vi "freq_scan_FRXYPPhase_6_23_2025.vi"() -> ()   [LabVIEW 2010]
uses:
  <vilib>/Utility/file.llb/Write To Spreadsheet File (string).vi
  <vilib>/Utility/file.llb/Write To Spreadsheet File (DBL).vi
panel:
  in  "DC offset":ext format="%.3f"
  in  "?":enum32{"Amp v.s Freq", "X & Y v.s Freq"}(tab)
  in  "Unit":i8=1 min=0 max=2 step=1
  in  "Start Frequency":dbl=1.635 min=0.0 format="%.3f"
  in  "End Frequency":dbl=3.0 min=0.0 format="%.3f"
  in  "Step in Hz":dbl=1.0 min=0.0 format="%.2f"
  in  "Step interval in ms":u32=500
  in  "Sensitivity":u16(ring)=20 items=["2 nV/fA", "5 nV/fA", "10 nV/fA", "20 nV/fA", "50 nV/fA", "100 nV/fA", "200 nV/fA", "500 nV/fA", "1 uV/pA", "2 uV/pA", "5 uV/pA", "10 uV/pA", "20 uV/pA", "50 uV/pA", "100 uV/pA", "200 uV/pA", "500 uV/pA", "1 mV/nA", "2 mV/nA", "5 mV/nA", "10 mV/nA", "20 mV/nA", "50 mV/nA", "100 mV/nA", "200 mV/nA", "500 mV/nA", "1 V/uA"]
  in  "Detection Bandwidth":u16(ring)=7 items=["25 kHz", "8.33 kHz", "2.50 kHz", "833 Hz", "250 Hz", "83.3 Hz", "25 Hz", "8.33 Hz", "2.50 Hz", "0.833 Hz", "0.250 Hz", "0.0833 Hz", "0.025 Hz"]
  in  "Phase":dbl
  in  "Driving amp (0 Vrms:0)":cluster{ext, i32}={0.05, 0} {"?" items=["Vrms", "Vpp", "dBm"]; "?" format="%.3f"}
  out "freq":string="22749"
  out "amp":string="0.000175477"
  out "Amp vs Freq":cluster{dbl, dbl}[](graph)=[{21250.0, 6.10356e-05}, {21252.3, 0.000320436}, {21254.6, 0.00027466}, {21256.899999999998, 0.000175477}, {21259.199999999997, 0.000297548}, {21261.499999999996, 0.000343325}, {21263.799999999996, 0.000251772}, {21266.099999999995, 0.00027466}, {21268.399999999994, 0.000297548}, {21270.699999999993, 6.8665e-05}, {21272.999999999993, 0.000251772}, {21275.299999999992, 9.91826e-05}, {21277.59999999999, 0.000251772}, {21279.89999999999, 0.00027466}, {21282.19999999999, 3.81472e-05}, {21284.49999999999, 0.000366213}, {21286.79999999999, 0.00013733}, {21289.099999999988, 0.000144959}, {21291.399999999987, 0.000221253}, {21293.699999999986, 0.000328066}, {21295.999999999985, 0.000259401}, {21298.299999999985, 0.000236512}, {21300.599999999984, 0.000228883}, {21302.899999999983, 0.000167848}, {21305.199999999983, 0.000297548}, {21307.49999999998, 0.000167848}, {21309.79999999998, 0.000213624}, {21312.09999999998, 0.000228883}, {21314.39999999998, 0.000289919}, {21316.69999999998, 0.00013733}, {21318.999999999978, 6.8665e-05}, {21321.299999999977, 0.000366213}, {21323.599999999977, 7.62944e-05}, {21325.899999999976, 0.000228883}, {21328.199999999975, 0.000381472}, {21330.499999999975, 0.000259401}, {21332.799999999974, 0.000167848}, {21335.099999999973, 0.000175477}, {21337.399999999972, 0.000343325}, {21339.69999999997, 0.000312807}, {21341.99999999997, 6.10356e-05}, {21344.29999999997, 0.000205995}, {21346.59999999997, 0.000129701}, {21348.89999999997, 0.000343325}, {21351.199999999968, 9.91826e-05}, {21353.499999999967, 0.000434877}, {21355.799999999967, 0.000373842}, {21358.099999999966, 0.000251772}, {21360.399999999965, 0.000328066}, {21362.699999999964, 0.000122071}, {21364.999999999964, 0.00039673}, {21367.299999999963, 0.000244142}, {21369.599999999962, 0.000366213}, {21371.89999999996, 0.000381472}, {21374.19999999996, 0.000350954}, {21376.49999999996, 0.000289919}, {21378.79999999996, 4.57766e-05}, {21381.09999999996, 0.000373842}, {21383.399999999958, 0.000312807}, {21385.699999999957, 9.91826e-05}, {21387.999999999956, 0.000114441}, {21390.299999999956, 0.000305178}, {21392.599999999955, 0.000175477}, {21394.899999999954, 0.000205995}, {21397.199999999953, 0.000190736}, {21399.499999999953, 0.00040436}, {21401.799999999952, 0.00013733}, {21404.09999999995, 9.91826e-05}, {21406.39999999995, 0.000320436}, {21408.69999999995, 0.000160218}, {21410.99999999995, 0.000419619}, {21413.29999999995, 0.000152589}, {21415.599999999948, 0.000320436}, {21417.899999999947, 0.000175477}, {21420.199999999946, 0.000183106}, {21422.499999999945, 9.91826e-05}, {21424.799999999945, 0.000152589}, {21427.099999999944, 0.000411989}, {21429.399999999943, 0.000366213}, {21431.699999999943, 0.000457766}, {21433.99999999994, 0.00040436}, {21436.29999999994, 0.000419619}, {21438.59999999994, 0.000259401}, {21440.89999999994, 0.000457766}, {21443.19999999994, 0.000205995}, {21445.499999999938, 0.000419619}, {21447.799999999937, 0.000106812}, {21450.099999999937, 0.000305178}, {21452.399999999936, 0.000267031}, {21454.699999999935, 0.00040436}, {21456.999999999935, 0.000381472}, {21459.299999999934, 0.000366213}, {21461.599999999933, 0.000411989}, {21463.899999999932, 0.000160218}, {21466.19999999993, 0.000259401}, {21468.49999999993, 0.000205995}, {21470.79999999993, 0.000282289}, {21473.09999999993, 0.000335695}, {21475.39999999993, 0.000328066}, {21477.699999999928, 0.000175477}, {21479.999999999927, 0.000419619}, {21482.299999999927, 0.00040436}, {21484.599999999926, 0.00040436}, {21486.899999999925, 0.000259401}, {21489.199999999924, 0.000236512}, {21491.499999999924, 0.000427248}, {21493.799999999923, 0.00039673}, {21496.099999999922, 0.000236512}, {21498.39999999992, 0.000373842}, {21500.69999999992, 0.000221253}, {21502.99999999992, 0.000465395}, {21505.29999999992, 0.000419619}, {21507.59999999992, 0.000320436}, {21509.899999999918, 0.000190736}, {21512.199999999917, 0.000465395}, {21514.499999999916, 0.000343325}, {21516.799999999916, 0.000473024}, {21519.099999999915, 0.000282289}, {21521.399999999914, 0.000419619}, {21523.699999999913, 0.000335695}, {21525.999999999913, 0.000411989}, {21528.299999999912, 0.000267031}, {21530.59999999991, 0.000289919}, {21532.89999999991, 0.000389101}, {21535.19999999991, 0.000236512}, {21537.49999999991, 0.000221253}, {21539.79999999991, 0.000450136}, {21542.099999999908, 0.000541691}, {21544.399999999907, 0.00039673}, {21546.699999999906, 0.000312807}, {21548.999999999905, 0.000205995}, {21551.299999999905, 0.000534061}, {21553.599999999904, 0.000442507}, {21555.899999999903, 0.000457766}, {21558.199999999903, 0.000434877}, {21560.4999999999, 0.000419619}, {21562.7999999999, 0.00039673}, {21565.0999999999, 0.000350954}, {21567.3999999999, 0.000534061}, {21569.6999999999, 0.000534061}, {21571.999999999898, 0.000328066}, {21574.299999999897, 0.000267031}, {21576.599999999897, 0.000564579}, {21578.899999999896, 0.000251772}, {21581.199999999895, 0.000541691}, {21583.499999999894, 0.000564579}, {21585.799999999894, 0.000579838}, {21588.099999999893, 0.000366213}, {21590.399999999892, 0.000343325}, {21592.69999999989, 0.000579838}, {21594.99999999989, 0.000579838}, {21597.29999999989, 0.000633243}, {21599.59999999989, 0.000480654}, {21601.89999999989, 0.000511173}, {21604.199999999888, 0.000488285}, {21606.499999999887, 0.000656132}, {21608.799999999886, 0.000366213}, {21611.099999999886, 0.000419619}, {21613.399999999885, 0.00067902}, {21615.699999999884, 0.000366213}, {21617.999999999884, 0.00039673}, {21620.299999999883, 0.00067139}, {21622.599999999882, 0.000633243}, {21624.89999999988, 0.000495914}, {21627.19999999988, 0.000427248}, {21629.49999999988, 0.00055695}, {21631.79999999988, 0.000427248}, {21634.09999999988, 0.00040436}, {21636.399999999878, 0.000579838}, {21638.699999999877, 0.000526432}, {21640.999999999876, 0.00067139}, {21643.299999999876, 0.000473024}, {21645.599999999875, 0.000610355}, {21647.899999999874, 0.000511173}, {21650.199999999873, 0.000526432}, {21652.499999999873, 0.000762943}, {21654.799999999872, 0.000762943}, {21657.09999999987, 0.000785831}, {21659.39999999987, 0.000595096}, {21661.69999999987, 0.000740055}, {21663.99999999987, 0.00080109}, {21666.29999999987, 0.000747684}, {21668.599999999868, 0.000564579}, {21670.899999999867, 0.000732426}, {21673.199999999866, 0.000602726}, {21675.499999999865, 0.00080872}, {21677.799999999865, 0.000656132}, {21680.099999999864, 0.000938419}, {21682.399999999863, 0.000846867}, {21684.699999999862, 0.000587467}, {21686.99999999986, 0.000709537}, {21689.29999999986, 0.000869755}, {21691.59999999986, 0.00067902}, {21693.89999999986, 0.000900272}, {21696.19999999986, 0.00067902}, {21698.499999999858, 0.000701908}, {21700.799999999857, 0.000999458}, {21703.099999999857, 0.000968937}, {21705.399999999856, 0.000885013}, {21707.699999999855, 0.00102998}, {21709.999999999854, 0.000839237}, {21712.299999999854, 0.000968937}, {21714.599999999853, 0.000823978}, {21716.899999999852, 0.000968937}, {21719.19999999985, 0.000991829}, {21721.49999999985, 0.00115968}, {21723.79999999985, 0.00114442}, {21726.09999999985, 0.00115968}, {21728.39999999985, 0.000999458}, {21730.699999999848, 0.000999458}, {21732.999999999847, 0.00110627}, {21735.299999999846, 0.000999458}, {21737.599999999846, 0.000938419}, {21739.899999999845, 0.00106812}, {21742.199999999844, 0.00126649}, {21744.499999999844, 0.00119019}, {21746.799999999843, 0.00110627}, {21749.099999999842, 0.00141145}, {21751.39999999984, 0.00105286}, {21753.69999999984, 0.00122071}, {21755.99999999984, 0.00141145}, {21758.29999999984, 0.001297}, {21760.59999999984, 0.00121308}, {21762.899999999838, 0.00139619}, {21765.199999999837, 0.00127412}, {21767.499999999836, 0.0014267}, {21769.799999999836, 0.00122071}, {21772.099999999835, 0.00154115}, {21774.399999999834, 0.00148011}, {21776.699999999833, 0.00144959}, {21778.999999999833, 0.00144196}, {21781.299999999832, 0.00157929}, {21783.59999999983, 0.00154877}, {21785.89999999983, 0.0016327}, {21788.19999999983, 0.0013733}, {21790.49999999983, 0.0016327}, {21792.79999999983, 0.00154115}, {21795.099999999828, 0.00177003}, {21797.399999999827, 0.00159455}, {21799.699999999826, 0.00157929}, {21801.999999999825, 0.0018921}, {21804.299999999825, 0.00180817}, {21806.599999999824, 0.00199129}, {21808.899999999823, 0.0018158}, {21811.199999999822, 0.00175477}, {21813.49999999982, 0.0020218}, {21815.79999999982, 0.00197603}, {21818.09999999982, 0.00199129}, {21820.39999999982, 0.00189973}, {21822.69999999982, 0.0019455}, {21824.999999999818, 0.00215913}, {21827.299999999817, 0.00206758}, {21829.599999999817, 0.0020981}, {21831.899999999816, 0.00238039}, {21834.199999999815, 0.00229646}, {21836.499999999814, 0.00234987}, {21838.799999999814, 0.00221254}, {21841.099999999813, 0.00251009}, {21843.399999999812, 0.00250246}, {21845.69999999981, 0.00238802}, {21847.99999999981, 0.00263979}, {21850.29999999981, 0.00263979}, {21852.59999999981, 0.00271608}, {21854.89999999981, 0.00264741}, {21857.199999999808, 0.00276949}, {21859.499999999807, 0.00289918}, {21861.799999999806, 0.00279237}, {21864.099999999806, 0.00311281}, {21866.399999999805, 0.00309755}, {21868.699999999804, 0.003006}, {21870.999999999804, 0.00324251}, {21873.299999999803, 0.00321962}, {21875.599999999802, 0.00341035}, {21877.8999999998, 0.00349428}, {21880.1999999998, 0.00351717}, {21882.4999999998, 0.00358583}, {21884.7999999998, 0.00382997}, {21887.0999999998, 0.00371553}, {21889.399999999798, 0.00389864}, {21891.699999999797, 0.0040665}, {21893.999999999796, 0.00415805}, {21896.299999999796, 0.00434116}, {21898.599999999795, 0.00444797}, {21900.899999999794, 0.00473788}, {21903.199999999793, 0.00467685}, {21905.499999999793, 0.00499728}, {21907.799999999792, 0.00508884}, {21910.09999999979, 0.00527957}, {21912.39999999979, 0.00547031}, {21914.69999999979, 0.00560763}, {21916.99999999979, 0.0060654}, {21919.29999999979, 0.00611117}, {21921.599999999788, 0.00637057}, {21923.899999999787, 0.00639346}, {21926.199999999786, 0.00661471}, {21928.499999999785, 0.007103}, {21930.799999999785, 0.00733188}, {21933.099999999784, 0.00738528}, {21935.399999999783, 0.00758365}, {21937.699999999782, 0.00788122}, {21939.99999999978, 0.00812536}, {21942.29999999978, 0.00841528}, {21944.59999999978, 0.00881201}, {21946.89999999978, 0.00908667}, {21949.19999999978, 0.00920874}, {21951.499999999778, 0.00949866}, {21953.799999999777, 0.00976568}, {21956.099999999777, 0.00971991}, {21958.399999999776, 0.0100632}, {21960.699999999775, 0.00996405}, {21962.999999999774, 0.0100861}, {21965.299999999774, 0.0105668}, {21967.599999999773, 0.0105591}, {21969.899999999772, 0.0102311}, {21972.19999999977, 0.0103455}, {21974.49999999977, 0.0102921}, {21976.79999999977, 0.00994879}, {21979.09999999977, 0.0101548}, {21981.39999999977, 0.00997931}, {21983.699999999768, 0.00973517}, {21985.999999999767, 0.00996405}, {21988.299999999766, 0.00971991}, {21990.599999999766, 0.00950629}, {21992.899999999765, 0.00929266}, {21995.199999999764, 0.00900275}, {21997.499999999764, 0.00892645}, {21999.799999999763, 0.00866705}, {22002.099999999762, 0.00841528}, {22004.39999999976, 0.00823981}, {22006.69999999976, 0.00823218}, {22008.99999999976, 0.00795752}, {22011.29999999976, 0.00795752}, {22013.59999999976, 0.00768283}, {22015.899999999758, 0.00753024}, {22018.199999999757, 0.00725558}, {22020.499999999756, 0.00695804}, {22022.799999999756, 0.00716403}, {22025.099999999755, 0.00704196}, {22027.399999999754, 0.00678256}, {22029.699999999753, 0.00693515}, {22031.999999999753, 0.00656894}, {22034.299999999752, 0.00638583}, {22036.59999999975, 0.00646213}, {22038.89999999975, 0.00610355}, {22041.19999999975, 0.00594333}, {22043.49999999975, 0.00572208}, {22045.79999999975, 0.00559238}, {22048.099999999748, 0.00569919}, {22050.399999999747, 0.00543979}, {22052.699999999746, 0.00527957}, {22054.999999999745, 0.00548556}, {22057.299999999745, 0.00524142}, {22059.599999999744, 0.00514987}, {22061.899999999743, 0.00496677}, {22064.199999999742, 0.00514224}, {22066.49999999974, 0.00485232}, {22068.79999999974, 0.00475314}, {22071.09999999974, 0.00464633}, {22073.39999999974, 0.004509}, {22075.69999999974, 0.00459293}, {22077.999999999738, 0.00452426}, {22080.299999999737, 0.00453189}, {22082.599999999737, 0.00426486}, {22084.899999999736, 0.00421146}, {22087.199999999735, 0.00408939}, {22089.499999999734, 0.00405887}, {22091.799999999734, 0.0039902}, {22094.099999999733, 0.0038376}, {22096.399999999732, 0.00404361}, {22098.69999999973, 0.00389864}, {22100.99999999973, 0.00384523}, {22103.29999999973, 0.00360109}, {22105.59999999973, 0.00365449}, {22107.89999999973, 0.00374605}, {22110.199999999728, 0.00364687}, {22112.499999999727, 0.00337984}, {22114.799999999726, 0.00334169}, {22117.099999999726, 0.00337984}, {22119.399999999725, 0.0035782}, {22121.699999999724, 0.0034485}, {22123.999999999724, 0.00320436}, {22126.299999999723, 0.00312807}, {22128.599999999722, 0.00314333}, {22130.89999999972, 0.00306703}, {22133.19999999972, 0.00307466}, {22135.49999999972, 0.00319673}, {22137.79999999972, 0.00307466}, {22140.09999999972, 0.00303651}, {22142.399999999718, 0.00295259}, {22144.699999999717, 0.00297548}, {22146.999999999716, 0.00293733}, {22149.299999999716, 0.00272371}, {22151.599999999715, 0.00291444}, {22153.899999999714, 0.00256349}, {22156.199999999713, 0.00259401}, {22158.499999999713, 0.00244142}, {22160.799999999712, 0.00264741}, {22163.09999999971, 0.00246431}, {22165.39999999971, 0.00253297}, {22167.69999999971, 0.00250246}, {22169.99999999971, 0.00232698}, {22172.29999999971, 0.0024872}, {22174.599999999708, 0.00251772}, {22176.899999999707, 0.00232698}, {22179.199999999706, 0.00205232}, {22181.499999999705, 0.00231935}, {22183.799999999705, 0.00214387}, {22186.099999999704, 0.00216676}, {22188.399999999703, 0.00218202}, {22190.699999999702, 0.00189973}, {22192.9999999997, 0.0021515}, {22195.2999999997, 0.00204469}, {22197.5999999997, 0.00198366}, {22199.8999999997, 0.00209047}, {22202.1999999997, 0.00180054}, {22204.499999999698, 0.00198366}, {22206.799999999697, 0.00195314}, {22209.099999999697, 0.00167847}, {22211.399999999696, 0.00170136}, {22213.699999999695, 0.00182343}, {22215.999999999694, 0.00162507}, {22218.299999999694, 0.00154115}, {22220.599999999693, 0.00186921}, {22222.899999999692, 0.001503}, {22225.19999999969, 0.00157166}, {22227.49999999969, 0.00162507}, {22229.79999999969, 0.00167084}, {22232.09999999969, 0.00130463}, {22234.39999999969, 0.00153352}, {22236.699999999688, 0.00160981}, {22238.999999999687, 0.00147248}, {22241.299999999686, 0.00160218}, {22243.599999999686, 0.00138093}, {22245.899999999685, 0.00153352}, {22248.199999999684, 0.00130463}, {22250.499999999683, 0.00126649}, {22252.799999999683, 0.00146485}, {22255.099999999682, 0.00121308}, {22257.39999999968, 0.00131989}, {22259.69999999968, 0.00119019}, {22261.99999999968, 0.00121308}, {22264.29999999968, 0.00110627}, {22266.59999999968, 0.00105286}, {22268.899999999678, 0.00122071}, {22271.199999999677, 0.00130463}, {22273.499999999676, 0.00130463}, {22275.799999999675, 0.00112153}, {22278.099999999675, 0.0011673}, {22280.399999999674, 0.00104523}, {22282.699999999673, 0.00134278}, {22284.999999999673, 0.00112916}, {22287.299999999672, 0.00126649}, {22289.59999999967, 0.00122071}, {22291.89999999967, 0.00103761}, {22294.19999999967, 0.00120545}, {22296.49999999967, 0.00128175}, {22298.79999999967, 0.00121308}, {22301.099999999667, 0.00110627}, {22303.399999999667, 0.00093079}, {22305.699999999666, 0.000953678}, {22307.999999999665, 0.0011673}, {22310.299999999665, 0.00110627}, {22312.599999999664, 0.00110627}, {22314.899999999663, 0.00121308}, {22317.199999999662, 0.00113679}, {22319.49999999966, 0.00117493}, {22321.79999999966, 0.00120545}, {22324.09999999966, 0.000961307}, {22326.39999999966, 0.000946049}, {22328.69999999966, 0.00128938}, {22330.999999999658, 0.00104523}, {22333.299999999657, 0.00102235}, {22335.599999999657, 0.00115968}, {22337.899999999656, 0.0012436}, {22340.199999999655, 0.00121308}, {22342.499999999654, 0.00120545}, {22344.799999999654, 0.00097657}, {22347.099999999653, 0.00108338}, {22349.399999999652, 0.00114442}, {22351.69999999965, 0.0011673}, {22353.99999999965, 0.00105286}, {22356.29999999965, 0.00097657}, {22358.59999999965, 0.00103761}, {22360.89999999965, 0.00131989}, {22363.199999999648, 0.0011673}, {22365.499999999647, 0.00127412}, {22367.799999999646, 0.00108338}, {22370.099999999646, 0.00121308}, {22372.399999999645, 0.00100709}, {22374.699999999644, 0.000999458}, {22376.999999999643, 0.00119019}, {22379.299999999643, 0.00119019}, {22381.599999999642, 0.00109101}, {22383.89999999964, 0.00125123}, {22386.19999999964, 0.00128175}, {22388.49999999964, 0.00105286}, {22390.79999999964, 0.00097657}, {22393.09999999964, 0.00130463}, {22395.399999999638, 0.00109864}, {22397.699999999637, 0.00104523}, {22399.999999999636, 0.00125123}, {22402.299999999635, 0.000869755}, {22404.599999999635, 0.00106812}, {22406.899999999634, 0.00117493}, {22409.199999999633, 0.000938419}, {22411.499999999633, 0.00122071}, {22413.799999999632, 0.00093079}, {22416.09999999963, 0.00107575}, {22418.39999999963, 0.00101472}, {22420.69999999963, 0.0011673}, {22422.99999999963, 0.00100709}, {22425.29999999963, 0.00118256}, {22427.599999999627, 0.00113679}, {22429.899999999627, 0.00101472}, {22432.199999999626, 0.00109101}, {22434.499999999625, 0.00112916}, {22436.799999999625, 0.00092316}, {22439.099999999624, 0.000839237}, {22441.399999999623, 0.00128175}, {22443.699999999622, 0.00121308}, {22445.99999999962, 0.00105286}, {22448.29999999962, 0.00109864}, {22450.59999999962, 0.00110627}, {22452.89999999962, 0.000823978}, {22455.19999999962, 0.000854496}, {22457.499999999618, 0.00103761}, {22459.799999999617, 0.00105286}, {22462.099999999617, 0.00097657}, {22464.399999999616, 0.000999458}, {22466.699999999615, 0.00102998}, {22468.999999999614, 0.000793461}, {22471.299999999614, 0.000732426}, {22473.599999999613, 0.00097657}, {22475.899999999612, 0.00102235}, {22478.19999999961, 0.000915531}, {22480.49999999961, 0.00097657}, {22482.79999999961, 0.000907902}, {22485.09999999961, 0.000823978}, {22487.39999999961, 0.00092316}, {22489.699999999608, 0.000831608}, {22491.999999999607, 0.000892643}, {22494.299999999606, 0.000732426}, {22496.599999999606, 0.000839237}, {22498.899999999605, 0.000709537}, {22501.199999999604, 0.000892643}, {22503.499999999603, 0.000793461}, {22505.799999999603, 0.000793461}, {22508.099999999602, 0.000854496}, {22510.3999999996, 0.000740055}, {22512.6999999996, 0.000877384}, {22514.9999999996, 0.000877384}, {22517.2999999996, 0.000526432}, {22519.5999999996, 0.000610355}, {22521.899999999598, 0.000770573}, {22524.199999999597, 0.000503544}, {22526.499999999596, 0.000816349}, {22528.799999999595, 0.000534061}, {22531.099999999595, 0.000717167}, {22533.399999999594, 0.000625614}, {22535.699999999593, 0.000656132}, {22537.999999999593, 0.000663761}, {22540.29999999959, 0.000434877}, {22542.59999999959, 0.000625614}, {22544.89999999959, 0.000473024}, {22547.19999999959, 0.000442507}, {22549.49999999959, 0.000717167}, {22551.799999999588, 0.00080109}, {22554.099999999587, 0.000350954}, {22556.399999999587, 0.000610355}, {22558.699999999586, 0.000526432}, {22560.999999999585, 0.000656132}, {22563.299999999585, 0.000633243}, {22565.599999999584, 0.000473024}, {22567.899999999583, 0.000328066}, {22570.199999999582, 0.00067139}, {22572.49999999958, 0.000564579}, {22574.79999999958, 0.000701908}, {22577.09999999958, 0.000526432}, {22579.39999999958, 0.000480654}, {22581.69999999958, 0.000656132}, {22583.999999999578, 0.00054932}, {22586.299999999577, 0.000381472}, {22588.599999999577, 0.000350954}, {22590.899999999576, 0.000511173}, {22593.199999999575, 0.000373842}, {22595.499999999574, 0.00027466}, {22597.799999999574, 0.000541691}, {22600.099999999573, 0.000663761}, {22602.399999999572, 0.000366213}, {22604.69999999957, 0.000564579}, {22606.99999999957, 0.00027466}, {22609.29999999957, 0.000511173}, {22611.59999999957, 0.00055695}, {22613.89999999957, 0.000312807}, {22616.199999999568, 0.000473024}, {22618.499999999567, 0.000473024}, {22620.799999999566, 0.000572208}, {22623.099999999566, 0.000465395}, {22625.399999999565, 0.000579838}, {22627.699999999564, 0.000465395}, {22629.999999999563, 0.000473024}, {22632.299999999563, 0.000427248}, {22634.599999999562, 0.00039673}, {22636.89999999956, 0.000480654}, {22639.19999999956, 0.000465395}, {22641.49999999956, 0.000534061}, {22643.79999999956, 0.000518803}, {22646.09999999956, 0.000289919}, {22648.399999999558, 0.000442507}, {22650.699999999557, 0.000541691}, {22652.999999999556, 0.000526432}, {22655.299999999555, 0.000534061}, {22657.599999999555, 0.000473024}, {22659.899999999554, 0.000457766}, {22662.199999999553, 0.000167848}, {22664.499999999553, 0.000259401}, {22666.79999999955, 0.000480654}, {22669.09999999955, 0.000175477}, {22671.39999999955, 0.00040436}, {22673.69999999955, 0.000221253}, {22675.99999999955, 0.000457766}, {22678.299999999548, 0.000518803}, {22680.599999999547, 0.000312807}, {22682.899999999547, 0.000312807}, {22685.199999999546, 0.000427248}, {22687.499999999545, 0.000366213}, {22689.799999999545, 0.000473024}, {22692.099999999544, 0.000473024}, {22694.399999999543, 0.00040436}, {22696.699999999542, 0.000450136}, {22698.99999999954, 0.000144959}, {22701.29999999954, 0.000228883}, {22703.59999999954, 0.000457766}, {22705.89999999954, 0.000144959}, {22708.19999999954, 8.39238e-05}, {22710.499999999538, 0.000411989}, {22712.799999999537, 0.000442507}, {22715.099999999537, 0.000228883}, {22717.399999999536, 0.000465395}, {22719.699999999535, 0.000259401}, {22721.999999999534, 0.000389101}, {22724.299999999534, 0.000503544}, {22726.599999999533, 0.000183106}, {22728.899999999532, 0.000289919}, {22731.19999999953, 0.00013733}, {22733.49999999953, 0.000244142}, {22735.79999999953, 0.000305178}, {22738.09999999953, 0.000259401}, {22740.39999999953, 0.000427248}, {22742.699999999528, 0.000221253}, {22744.999999999527, 9.91826e-05}, {22747.299999999526, 0.000175477}]
  out "Waveform Chart":cluster{dbl, dbl}(graph)
  in  "Path":path
  in  "On/Off":bool=TRUE
  # "Make sure to set DS345's GPIB address to 19.\nMake sure to set SR830's GPIB address to 8."
  # "0: Hz\n1: kHz\n2: MHz"
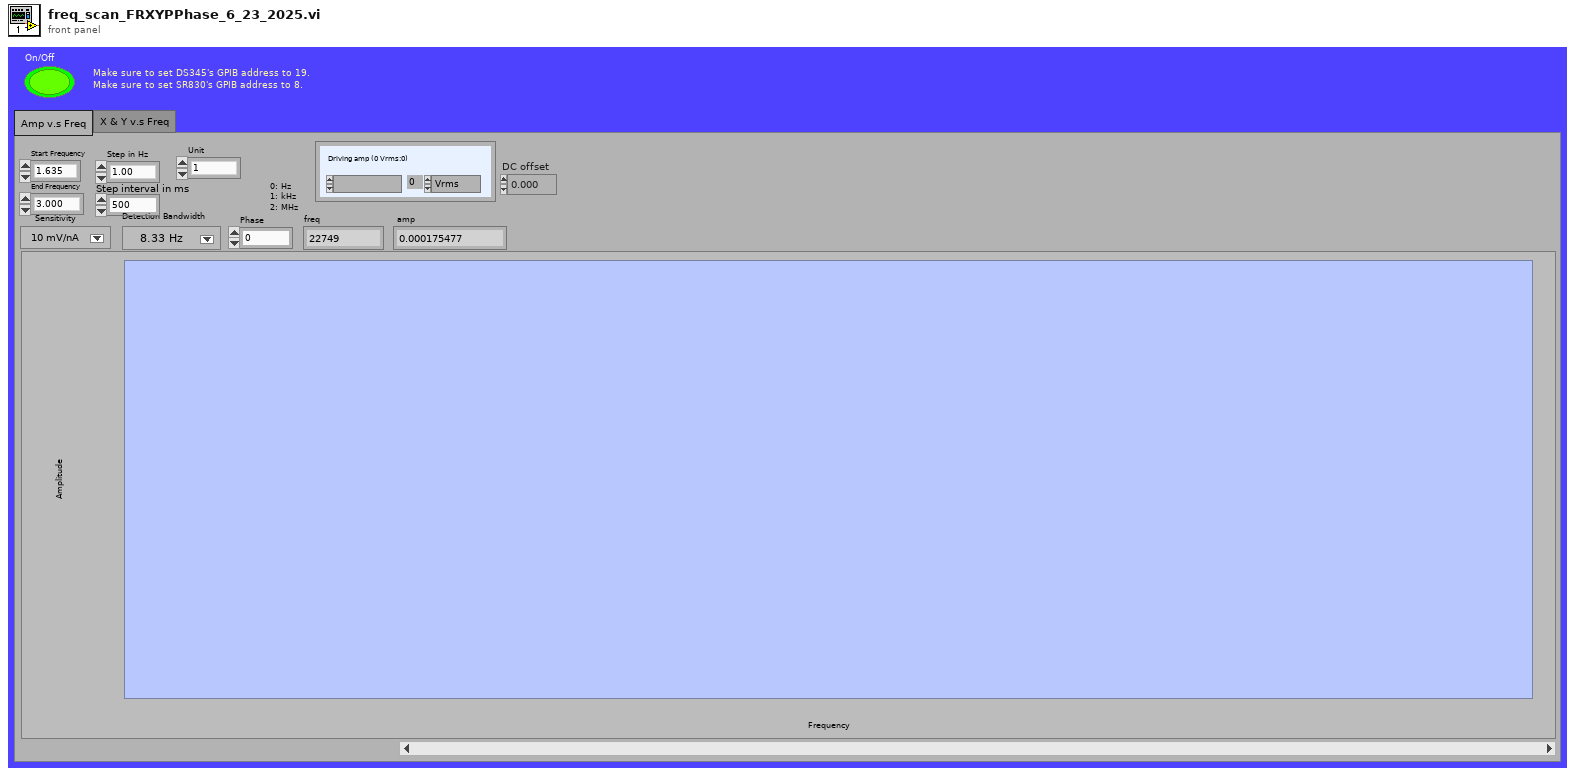
[diagram p1: front panel]
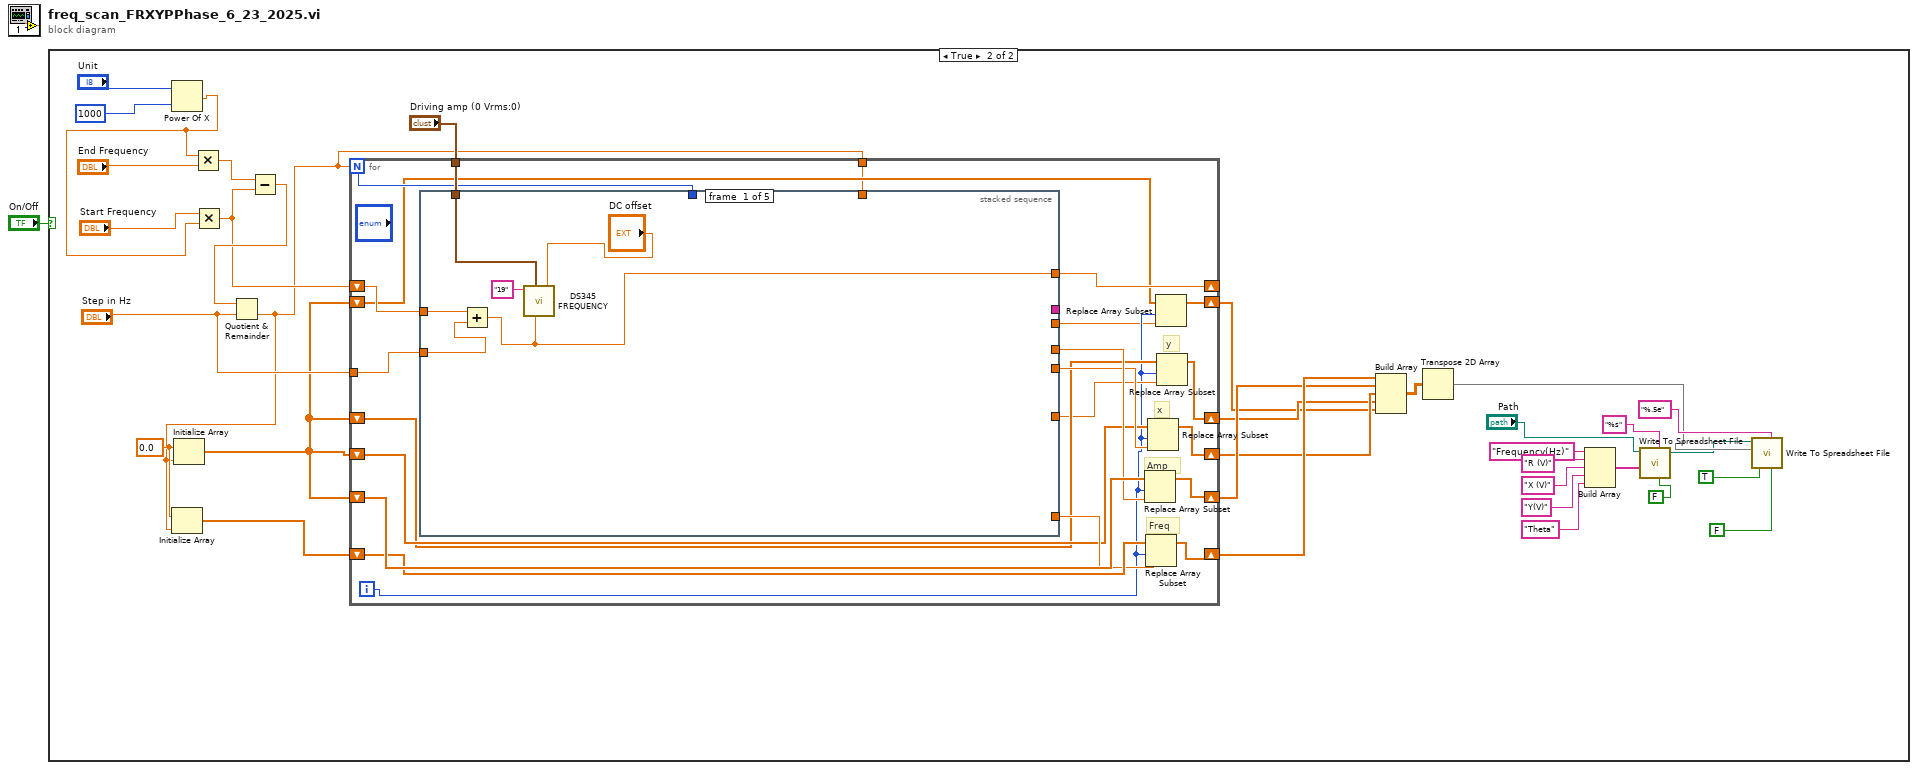
[diagram p0: block diagram]
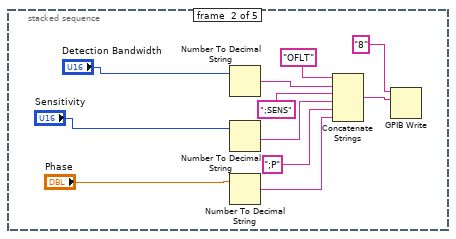
[diagram p3: hidden frame]
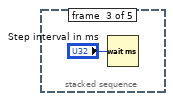
[diagram p4: hidden frame]
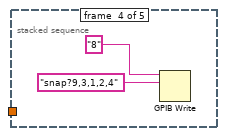
[diagram p5: hidden frame]
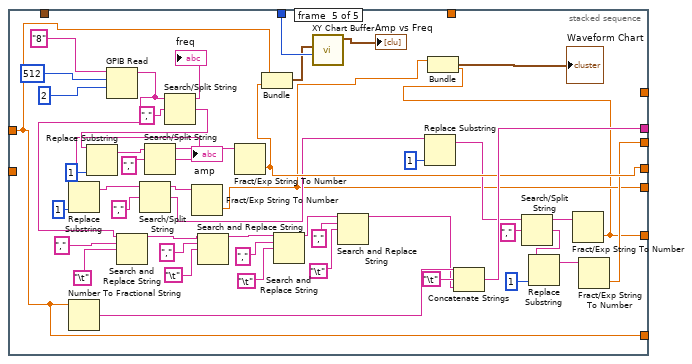
[diagram p6: hidden frame]
diagram:
  n1 = case shown="True" "On/Off" {
    frame False {
    }
    frame True {
      w25 = 0.0 ("element")
      n2 = Power Of X(1:1000, 2:"Unit") -> (0:w33:dbl)
      n3 = Multiply(x=w33, y="End Frequency") -> (x*y=w29:dbl)
      n4 = Multiply(x="Start Frequency", y=w33) -> (x*y=w28:dbl)
      n5 = Subtract(x=w29, y=w28) -> (x-y=w30:dbl)
      n6 = Quotient & Remainder(x=w30, y="Step in Hz") -> (floor(x/y)=w2:dbl)  [unwired: 1 out]
      n7 = Initialize Array(w25, w2) -> (w24:dbl[])
      n8 = Initialize Array(w25, w2) -> (w20:dbl[])
      n9 = for {
        N: w2 -> [w54]
        shift-right: [w41] -> _
        shift-left: w28 -> [w56]
        tunnel: "Step in Hz" -> [w57]
        tunnel: "Driving amp (0 Vrms:0)" -> [w55]
        shift-right: [w52] -> w18
        shift-left: w20 -> [w53]
        shift-right: [w49] -> w19
        shift-left: w24 -> [w51]
        shift-right: [w44] -> w17
        shift-left: w20 -> [w46]
        shift-right: [w42] -> w16
        shift-left: w20 -> [w45]
        shift-right: [w38] -> w15
        shift-left: w20 -> [w37]
        tunnel: w2 -> [w36]
        i -> [w40]
        # "Amp"
        # "Freq"
        # "x"
        # "y"
        n10 = stacked-sequence {
          tunnel: w57 -> [w61 _ _ _ _]
          tunnel: w56 -> [w63 _ _ _ w82]
          tunnel: [w62 _ _ _ _] -> w41
          tunnel: w55 -> [w59 _ _ _ _]
          tunnel: w54 -> [_ _ _ _ w120]
          tunnel: [_ _ _ _ w100] -> _
          tunnel: [_ _ _ _ w82] -> w50
          tunnel: [_ _ _ _ w98] -> w48
          tunnel: [_ _ _ _ w80] -> w47
          tunnel: [_ _ _ _ w79] -> w43
          tunnel: [_ _ _ _ w93] -> w39
          tunnel: w36 -> [_ _ _ _ _]
          frame #0 {
            n11 = Add(x=w63, y=w61) -> (x+y=w62:dbl)
            n12 = call "DS345 FREQUENCY.vi"("GPIB address"="19", "amplitude (0 Vrms:0)"=w59, "frequency"=w62, "DC offset"="DC offset") -> ()  [unwired: 4 in, 1 out]
          }
          frame #1 {
            n13 = Number To Decimal String(number="Detection Bandwidth") -> (decimal integer string=w73:string)  [unwired: 1 out]
            n14 = Number To Decimal String(number="Sensitivity") -> (decimal integer string=w71:string)  [unwired: 1 out]
            n15 = Number To Decimal String(number="Phase") -> (decimal integer string=w65:string)  [unwired: 1 out]
            n16 = Concatenate Strings("OFLT", w73, ";SENS", w71, ";P", w65) -> (w64:string)
            n17 = GPIB Write(0:"8" ("address string"), 1:w64) -> ()  [unwired: 1 in, 4 out]
          }
          frame #2 {
            n18 = Wait (ms)(milliseconds to wait="Step interval in ms") -> ()  [unwired: 1 out]
          }
          frame #3 {
            n19 = GPIB Write(0:"8" ("address string"), 1:"snap?9,3,1,2,4" ("data")) -> ()  [unwired: 1 in, 4 out]
          }
          frame #4 {
            n20 = Number To Fractional String(number=w82) -> (F-format string=w102:string)  [unwired: 3 out]
            n21 = GPIB Read(0:"8" ("address string"), 1:512 ("byte count"), 2:i16 2 ("mode (0)")) -> (5:w83:string)  [unwired: 1 in, 3 out]
            n22 = Search and Replace String(input string=w83, search string=",", replace string="\t") -> (result string=w111:string)  [unwired: 1 in, 7 out]
            n23 = Search/Split String(string=w83, search string/char (-)=",") -> (substring before match=→"freq":string, match + rest of string=w118:string)  [unwired: 2 out]
            n24 = Replace Substring(2:1 ("length (len. of substring)"), 5:w118) -> (1:w116:string)  [unwired: 3 out]
            n25 = Search/Split String(string=w116, search string/char (-)=",") -> (substring before match=w114:string, match + rest of string=w91:string)  [unwired: 2 out]
            "amp" <- w114
            n26 = Replace Substring(2:1, 5:w91) -> (1:w90:string)  [unwired: 3 out]
            n27 = Search/Split String(string=w90, search string/char (-)=",") -> (substring before match=w96:string, match + rest of string=w88:string)  [unwired: 2 out]
            n28 = Fract/Exp String To Number(string=w96) -> (number=w80:dbl)  [unwired: 4 out]
            n29 = Search and Replace String(input string=w111, search string=",", replace string="\t") -> (result string=w108:string)  [unwired: 1 in, 7 out]
            n30 = Fract/Exp String To Number(string=w114) -> (number=w98:dbl)  [unwired: 4 out]
            n31 = Bundle(w82, w98) -> (w81:cluster{dbl, dbl})  [unwired: 1 out]
            n32 = Search and Replace String(input string=w108, search string=",", replace string="\t") -> (result string=w105:string)  [unwired: 1 in, 7 out]
            n33 = call "XY Chart Buffer.vi"("chart length (points)"=w120, "new point"=w81) -> ("XY chart data"=→"Amp vs Freq":cluster{"x":dbl, "y":dbl}[])  [unwired: 2 in, 7 out]
            n34 = Search and Replace String(input string=w105, search string=",", replace string="\t") -> (result string=w99:string)  [unwired: 1 in, 7 out]
            n35 = Replace Substring(2:1, 5:w88) -> (1:w87:string)  [unwired: 3 out]
            n36 = Concatenate Strings(w102, "\t", w99) -> (w100:string)
            n37 = Search/Split String(string=w87, search string/char (-)=",") -> (substring before match=w94:string, match + rest of string=w86:string)  [unwired: 2 out]
            n38 = Replace Substring(2:1, 5:w86) -> (1:w84:string)  [unwired: 3 out]
            n39 = Fract/Exp String To Number(string=w94) -> (number=w79:dbl)  [unwired: 4 out]
            n40 = Bundle(w80, w79) -> (→"Waveform Chart":cluster{dbl, dbl})  [unwired: 1 in]
            n41 = Fract/Exp String To Number(string=w84) -> (number=w93:dbl)  [unwired: 4 out]
          }
        }
        n42 = Replace Array Subset(array=w53, new element=w48, index=w40) -> (w52:dbl[])
        n43 = Replace Array Subset(array=w51, new element=w50, index=w40) -> (w49:dbl[])
        n44 = Replace Array Subset(array=w46, new element=w47, index=w40) -> (w44:dbl[])
        n45 = Replace Array Subset(array=w37, new element=w39, index=w40) -> (w38:dbl[])
        n46 = Replace Array Subset(array=w45, new element=w43, index=w40) -> (w42:dbl[])
      }
      n47 = Build Array(w19, w18, w17, w16, w15) -> (w22:dbl[][])
      n48 = Transpose 2D Array(2D array=w22) -> (transposed array=w21:dbl[][])
      n49 = Build Array("Frequency(Hz)", "R (V)" ("element"), "X (V)" ("element"), "Y(V)" ("element"), "Theta" ("element")) -> (w9:string[])
      n50 = call-poly <vilib>:"Write To Spreadsheet File.vi"("transpose? (no:F)"=FALSE, "format (%s)"="%s" ("format (%.3f)"), "1D data"=w9, "file path (dialog if empty)"="Path") -> ("new file path (Not A Path if cancelled)"=w13:path)  [unwired: 2 in, 2 out]
      n51 = call-poly <vilib>:"Write To Spreadsheet File.vi"("transpose? (no:F)"=FALSE, "format (%.3f)"="%.5e", "append to file? (new file:F)"=TRUE, "2D data"=w21, "file path (dialog if empty)"=w13) -> ()  [unwired: 1 in, 3 out]
    }
  }
